vi "Windspeed Warnings.vi"(8 "错误输入":cluster{"状态":bool, "代码":i32, "源":string}, 11 "气象数据输入":T1={"当前温度"=0.0, "最高温度"=0.0, "最低温度"=0.0, "温度警告？"=FALSE, "温度警告文本"="无警告", "当前风速"=0.0, "最大风速"=0.0, "风速警告？"=FALSE, "风速警告文本"="无警告"}) -> (0 "错误输出":cluster{"状态":bool, "代码":i32, "源":string}, 3 "气象数据输出":T1={"当前温度"=0.0, "最高温度"=0.0, "最低温度"=0.0, "温度警告？"=FALSE, "温度警告文本"="无警告", "当前风速"=0.0, "最大风速"=0.0, "风速警告？"=FALSE, "风速警告文本"="无警告"})   [LabVIEW 2012]
doc: "本VI用于判定基于当前风速值和边界设置的字符串，该字符串输出至气象站。"
uses:
  Weather Data.ctl
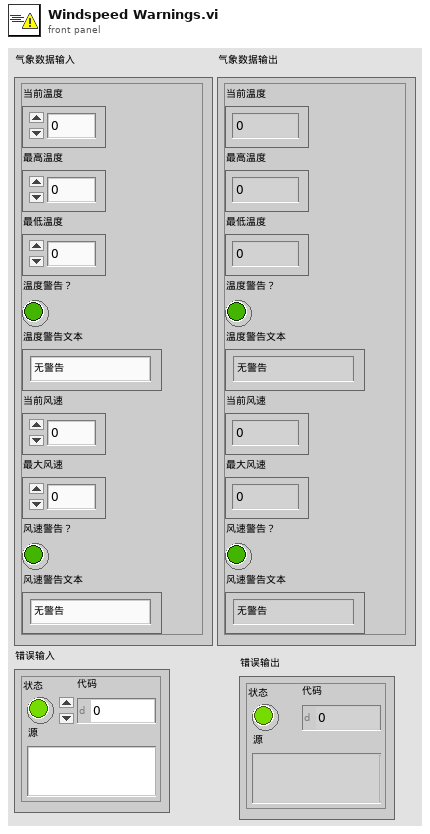
[diagram p1: front panel]
types:
  T1 = typedef "Weather Data.ctl" = cluster{"当前温度":dbl, "最高温度":dbl, "最低温度":dbl, "温度警告？":bool, "温度警告文本":string, "当前风速":dbl, "最大风速":dbl, "风速警告？":bool, "风速警告文本":string}
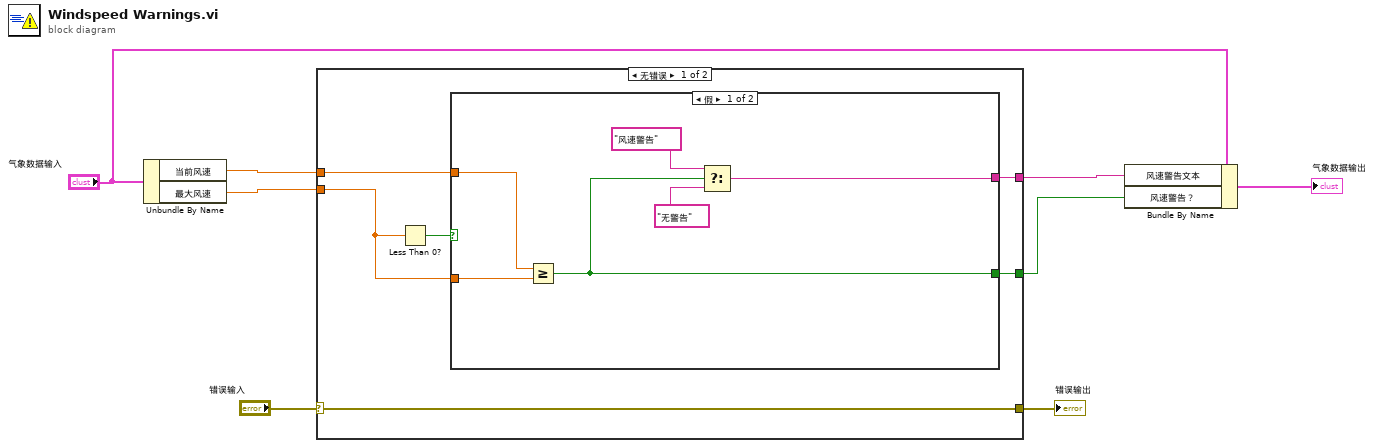
[diagram p0: block diagram]
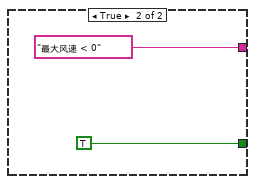
[diagram p2: hidden frame]
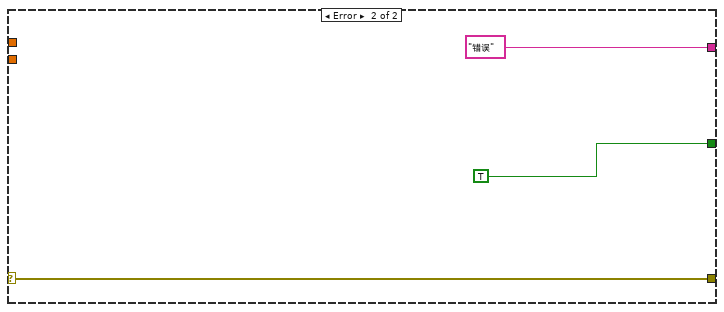
[diagram p3: hidden frame]
diagram:
  n1 = Unbundle By Name ("按名称解除捆绑")("气象数据输入") -> ("当前风速"=w6:dbl, "最大风速"=w5:dbl)
  n2 = case shown="无错误" "错误输入" {
    selector: "错误输入" -> [w11 w25]
    tunnel: [w14 "错误" ("f")] -> w3
    tunnel: [w13 TRUE] -> w2
    tunnel: [w11 w25] -> w7
    tunnel: w6 -> [w10 _]
    tunnel: w5 -> [w9 _]
    frame No Error {
      n3 = Less Than 0? ("小于0？")(x=w9) -> (x < 0?=w12:bool)
      n4 = case shown="假" w12 {
        tunnel: [w16 "最大风速 < 0" ("f")] -> w14
        tunnel: [w15 TRUE] -> w13
        tunnel: w9 -> [w20 _]
        tunnel: w10 -> [w17 _]
        frame False {
          n5 = Greater Or Equal? ("大于等于？")(x=w17, y=w20) -> (x >= y?=w15:bool)
          n6 = Select ("选择")(t="风速警告", s=w15, f="无警告") -> (s? t:f=w16:string)
        }
        frame True {
        }
      }
    }
    frame Error {
    }
  }
  "错误输出" <- w7
  n7 = Bundle By Name ("按名称捆绑")(cluster="气象数据输入", "风速警告文本"=w3, "风速警告？"=w2) -> (→"气象数据输出":T1)
